vi "ReadChannelDataVectors.vi"(0 "axis in":cluster{"keyHandle":u32, "nodeId":u16}={"keyHandle"=0, "nodeId"=1}, 5 "recorded objects":T1 {"recorded object 4"."objectSubIndex" format="%x"; "recorded object 4"."objectIndex" format="%x"; "recorded object 3"."objectSubIndex" format="%x"; "recorded object 3"."objectIndex" format="%x"; "recorded object 2"."objectSubIndex" format="%x"; "recorded object 2"."objectIndex" format="%x"; "recorded object 1"."objectSubIndex" format="%x"; "recorded object 1"."objectIndex" format="%x"}, 9 "waitBeforeRead":u32, 11 "error in (no error)":errorcluster) -> (4 "axis out":cluster{"keyHandle":u32, "nodeId":u16}={"keyHandle"=0, "nodeId"=1}, 6 "U8 data vectors":T2, 8 "U16 data vectors":cluster{u16[], u16[], u16[], u16[]}, 10 "U32 data vectors":cluster{u32[], u32[], u32[], u32[]}, 15 "error out":errorcluster)   [LabVIEW 2019, in "maxonEPOS.lvlib"]
doc: "<B>ReadChannelDataVectors</B> returns the data points of the recorded data channels."
uses:
  Examples/maxonEPOS.lvlib
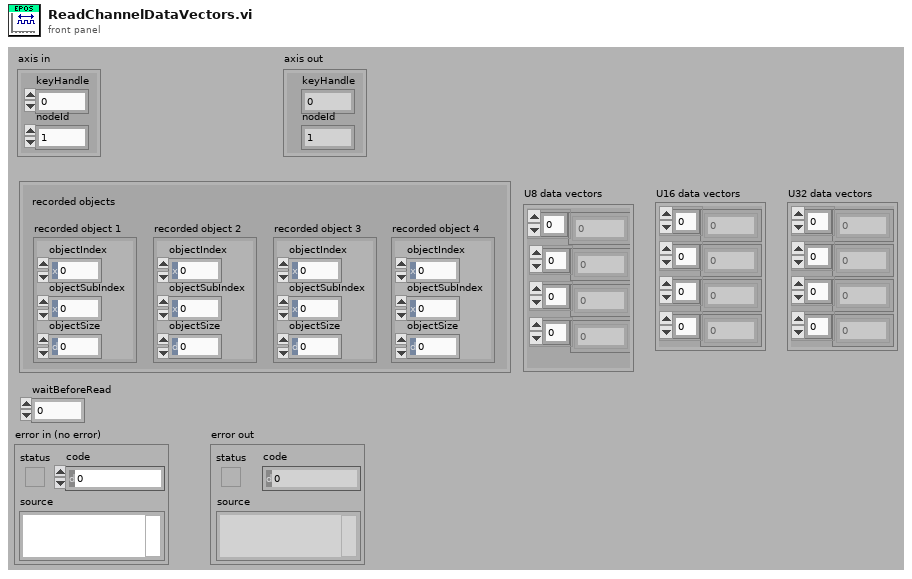
[diagram p1: front panel]
types:
  T1 = cluster{"recorded object 1":cluster{"objectIndex":u16, "objectSubIndex":u8, "objectSize":u8}, "recorded object 2":cluster{"objectIndex":u16, "objectSubIndex":u8, "objectSize":u8}, "recorded object 3":cluster{"objectIndex":u16, "objectSubIndex":u8, "objectSize":u8}, "recorded object 4":cluster{"objectIndex":u16, "objectSubIndex":u8, "objectSize":u8}}
  T2 = cluster{"data vector channel 1":u8[], "data vector channel 2":u8[], "data vector channel 3":u8[], "data vector channel 4":u8[]}
  T3 = cluster{"objectIndex":u16, "objectSubIndex":u8, "objectSize":u8}
  T4 = cluster{"data vector":u8[], "data vector":u8[], "data vector":u8[], "data vector":u8[]}
  T5 = cluster{"data vector buffer":u8[], "data vector buffer":u8[], "data vector buffer":u8[], "data vector buffer":u8[]}
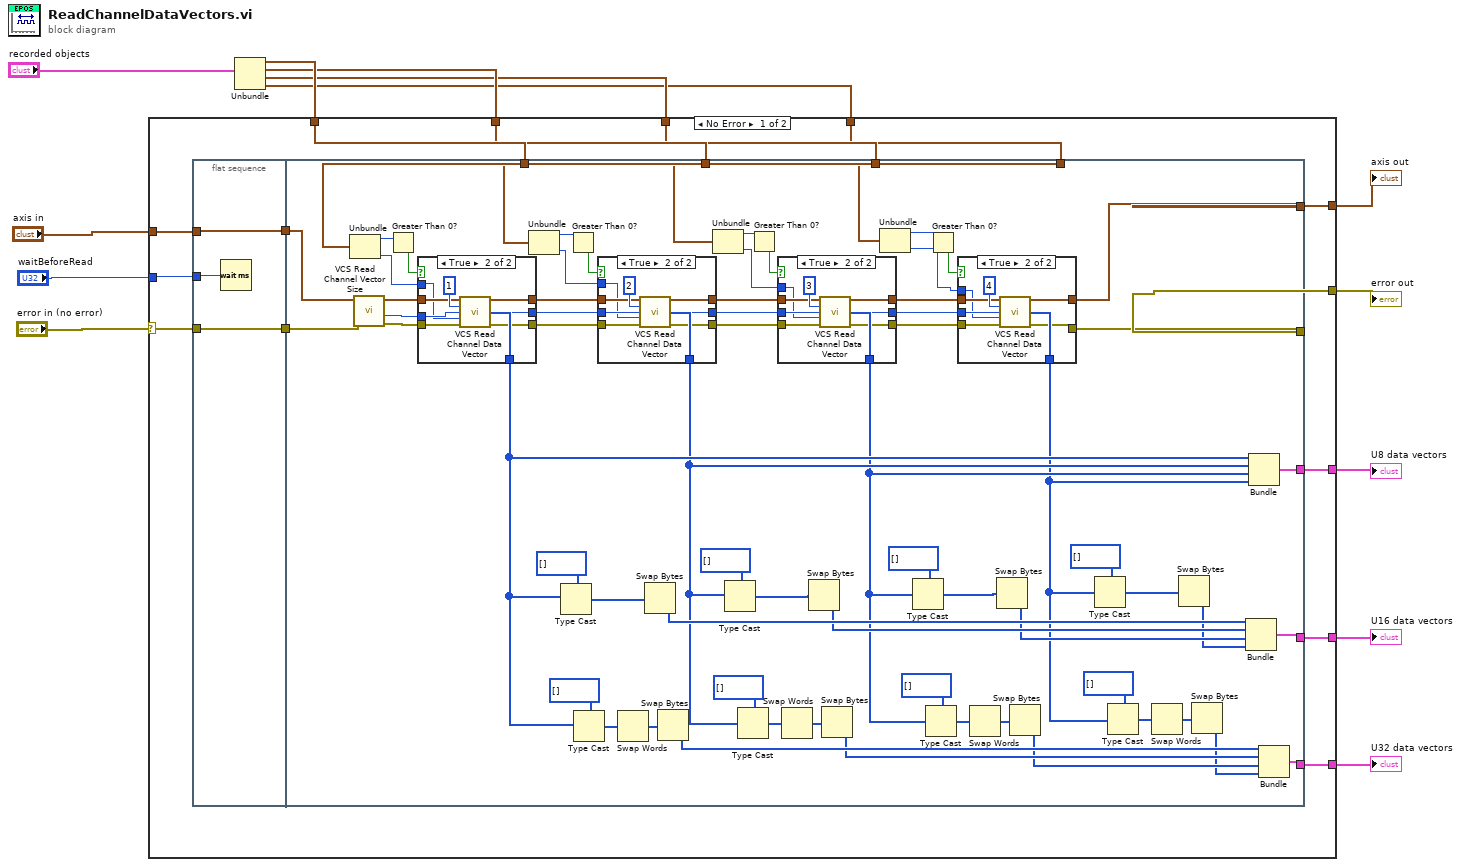
[diagram p0: block diagram]
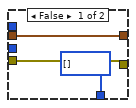
[diagram p2: hidden frame]
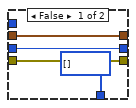
[diagram p3: hidden frame]
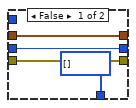
[diagram p4: hidden frame]
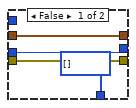
[diagram p5: hidden frame]
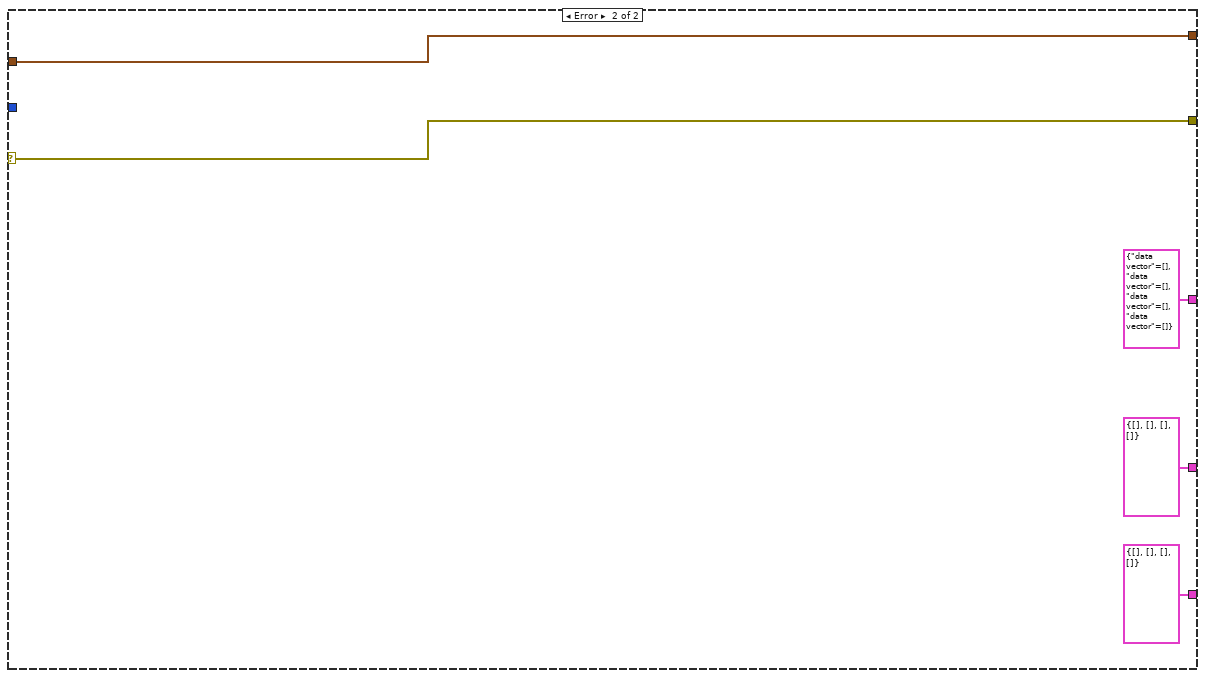
[diagram p6: hidden frame]
diagram:
  n1 = Unbundle("recorded objects") -> ("recorded object 1"=w8:T3, "recorded object 2"=w7:T3, "recorded object 3"=w6:T3, "recorded object 4"=w5:T3)
  n2 = case shown="No Error" "error in (no error)" {
    selector: "error in (no error)" -> [w19 w149]
    tunnel: [w18 w149] -> w12
    tunnel: [w17 w148] -> w11
    tunnel: "axis in" -> [w21 w148]
    tunnel: w8 -> [w27 _]
    tunnel: w7 -> [w26 _]
    tunnel: w6 -> [w25 _]
    tunnel: w5 -> [w24 _]
    tunnel: "waitBeforeRead" -> [w23 _]
    tunnel: [w16 T4 {"data vector"=[], "data vector"=[], "data vector"=[], "data vector"=[]}] -> w1
    tunnel: [w15 cluster{u32[], u32[], u32[], u32[]} {[], [], [], []}] -> w3
    tunnel: [w14 cluster{u16[], u16[], u16[], u16[]} {[], [], [], []}] -> w2
    frame No Error {
      n3 = flat-sequence {
        tunnel: w23 -> [w30]
        tunnel: [w29] -> w22
        tunnel: w21 -> [w29]
        tunnel: [w28] -> w20
        tunnel: w19 -> [w28]
        tunnel: w27 -> [w77]
        tunnel: w26 -> [w76]
        tunnel: w25 -> [w75]
        tunnel: w24 -> [w74]
        tunnel: w22 -> [w69]
        tunnel: w20 -> [w68]
        tunnel: [w67] -> w18
        tunnel: [w66] -> w17
        tunnel: [w65] -> w16
        tunnel: [w48] -> w15
        tunnel: [w35] -> w14
        frame #0 {
          n4 = Wait (ms)(milliseconds to wait=w30) -> ()  [unwired: 1 out]
        }
        frame #1 {
          n5 = Unbundle(w77) -> ("objectIndex"=w70:u16, "objectSize"=w94:u8)  [unwired: 1 out]
          n6 = call "VCS Read Channel Vector Size.vi"("error in (no error)"=w68, "axis in"=w69) -> ("error out"=w85:errorcluster, "vector size"=w86:u32, "axis out"=w84:cluster{"keyHandle":u32, "nodeId":u16})  [unwired: 7 in]
          n7 = Greater Than 0?(x=w70) -> (x > 0?=w90:bool)
          n8 = case shown="True" w90 {
            tunnel: [u8[] [] ("data vector") w143] -> w34
            tunnel: w84 -> [w136 w142]
            tunnel: [w136 w141] -> w78
            tunnel: w85 -> [w135 w140]
            tunnel: [w135 w139] -> w81
            tunnel: w86 -> [w133 w138]
            tunnel: [w133 w138] -> w87
            tunnel: w94 -> [_ w137]
            frame False {
            }
            frame True {
              n9 = call "VCS Read Channel Data Vector.vi"("axis in"=w142, "channelNumber"=u8 1, "vectorBufferSize"=w138, "objectSize"=w137, "error in (no error)"=w140) -> ("axis out"=w141:cluster{"keyHandle":u32, "nodeId":u16}, "data vector buffer"=w143:u8[], "error out"=w139:errorcluster)  [unwired: 8 in]
            }
          }
          n10 = Unbundle(w76) -> ("objectIndex"=w71:u16, "objectSize"=w95:u8)  [unwired: 1 out]
          n11 = Type Cast(type=u16[] [] ("Array"), x=w34) -> (*(type *) &x=w39:u16[])
          n12 = Greater Than 0?(x=w71) -> (x > 0?=w93:bool)
          n13 = Type Cast(type=u32[] [] ("Array"), x=w34) -> (*(type *) &x=w61:u32[])
          n14 = case shown="True" w93 {
            tunnel: [u8[] [] ("data vector") w131] -> w33
            tunnel: w78 -> [w124 w130]
            tunnel: [w124 w129] -> w79
            tunnel: w81 -> [w123 w128]
            tunnel: [w123 w127] -> w82
            tunnel: w87 -> [w121 w126]
            tunnel: [w121 w126] -> w88
            tunnel: w95 -> [_ w125]
            frame False {
            }
            frame True {
              n15 = call "VCS Read Channel Data Vector.vi"("axis in"=w130, "channelNumber"=u8 2, "vectorBufferSize"=w126, "objectSize"=w125, "error in (no error)"=w128) -> ("axis out"=w129:cluster{"keyHandle":u32, "nodeId":u16}, "data vector buffer"=w131:u8[], "error out"=w127:errorcluster)  [unwired: 8 in]
            }
          }
          n16 = Swap Words(1:w61) -> (0:w60:u32[])
          n17 = Swap Bytes(anything=w39) -> (byte swapped=w43:u16[])
          n18 = Swap Bytes(anything=w60) -> (byte swapped=w52:u32[])
          n19 = Unbundle(w75) -> ("objectIndex"=w73:u16, "objectSize"=w96:u8)  [unwired: 1 out]
          n20 = Type Cast(type=u16[] [] ("Array"), x=w33) -> (*(type *) &x=w38:u16[])
          n21 = Type Cast(type=u32[] [] ("Array"), x=w33) -> (*(type *) &x=w59:u32[])
          n22 = Greater Than 0?(x=w73) -> (x > 0?=w91:bool)
          n23 = case shown="True" w91 {
            tunnel: [u8[] [] ("data vector") w119] -> w32
            tunnel: w79 -> [w112 w118]
            tunnel: [w112 w117] -> w80
            tunnel: w82 -> [w111 w116]
            tunnel: [w111 w115] -> w83
            tunnel: w88 -> [w109 w114]
            tunnel: [w109 w114] -> w89
            tunnel: w96 -> [_ w113]
            frame False {
            }
            frame True {
              n24 = call "VCS Read Channel Data Vector.vi"("axis in"=w118, "channelNumber"=u8 3, "vectorBufferSize"=w114, "objectSize"=w113, "error in (no error)"=w116) -> ("axis out"=w117:cluster{"keyHandle":u32, "nodeId":u16}, "data vector buffer"=w119:u8[], "error out"=w115:errorcluster)  [unwired: 8 in]
            }
          }
          n25 = Swap Words(1:w59) -> (0:w58:u32[])
          n26 = Swap Bytes(anything=w38) -> (byte swapped=w42:u16[])
          n27 = Swap Bytes(anything=w58) -> (byte swapped=w51:u32[])
          n28 = Unbundle(w74) -> ("objectIndex"=w72:u16, "objectSize"=w97:u8)  [unwired: 1 out]
          n29 = Type Cast(type=u16[] [] ("Array"), x=w32) -> (*(type *) &x=w37:u16[])
          n30 = Type Cast(type=u32[] [] ("Array"), x=w32) -> (*(type *) &x=w57:u32[])
          n31 = Greater Than 0?(x=w72) -> (x > 0?=w92:bool)
          n32 = case shown="True" w92 {
            tunnel: [u8[] [] ("data vector") w107] -> w31
            tunnel: w80 -> [w100 w106]
            tunnel: [w100 w105] -> w66
            tunnel: w83 -> [w99 w104]
            tunnel: [w99 w103] -> w67
            tunnel: w89 -> [_ w102]
            tunnel: w97 -> [_ w101]
            frame False {
            }
            frame True {
              n33 = call "VCS Read Channel Data Vector.vi"("axis in"=w106, "channelNumber"=u8 4, "vectorBufferSize"=w102, "objectSize"=w101, "error in (no error)"=w104) -> ("axis out"=w105:cluster{"keyHandle":u32, "nodeId":u16}, "data vector buffer"=w107:u8[], "error out"=w103:errorcluster)  [unwired: 8 in]
            }
          }
          n34 = Swap Words(1:w57) -> (0:w56:u32[])
          n35 = Swap Bytes(anything=w37) -> (byte swapped=w41:u16[])
          n36 = Swap Bytes(anything=w56) -> (byte swapped=w50:u32[])
          n37 = Type Cast(type=u16[] [] ("Array"), x=w31) -> (*(type *) &x=w36:u16[])
          n38 = Type Cast(type=u32[] [] ("Array"), x=w31) -> (*(type *) &x=w54:u32[])
          n39 = Swap Words(1:w54) -> (0:w53:u32[])
          n40 = Swap Bytes(anything=w36) -> (byte swapped=w40:u16[])
          n41 = Swap Bytes(anything=w53) -> (byte swapped=w49:u32[])
          n42 = Bundle(w43, w42, w41, w40) -> (w35:cluster{u16[], u16[], u16[], u16[]})  [unwired: 1 in]
          n43 = Bundle("data vector buffer"=w34, "data vector buffer"=w33, "data vector buffer"=w32, "data vector buffer"=w31) -> (w65:T5)  [unwired: 1 in]
          n44 = Bundle(w52, w51, w50, w49) -> (w48:cluster{u32[], u32[], u32[], u32[]})  [unwired: 1 in]
        }
      }
    }
    frame Error {
    }
  }
  "error out" <- w12
  "axis out" <- w11
  "U8 data vectors" <- w1
  "U32 data vectors" <- w3
  "U16 data vectors" <- w2
